vi "Increment Current Index.vi"(8 "Error In":errorcluster, 11 "reference in":refnum<class "Recipe.lvclass">) -> (0 "Error Out":errorcluster, 3 "reference out":refnum<class "Recipe.lvclass">)   [LabVIEW 2021, in "Recipe.lvclass"]
uses:
  Recipe.lvclass
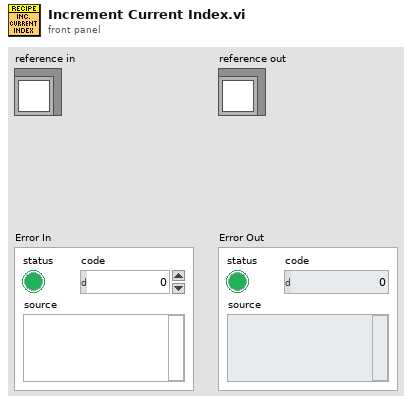
[diagram p1: front panel]
types:
  T1 = typedef "Recipe.lvclass/ObjectAttributes.ctl" = cluster{"Steps":refnum<class "Recipe Step.lvclass">[], "Current Info":cluster{"Current Index":u64}}
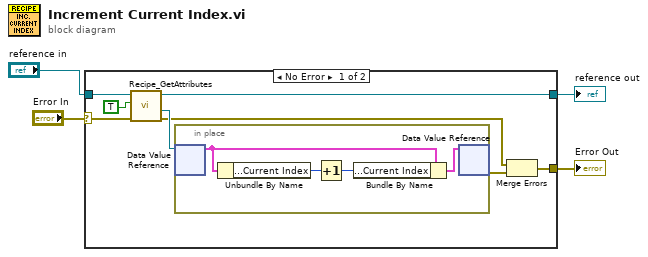
[diagram p0: block diagram]
diagram:
  n1 = case shown="No Error" "Error In" {
    selector: "Error In" -> [w11 w18]
    tunnel: [w8 w18] -> w3
    tunnel: [w9 w17] -> w1
    tunnel: "reference in" -> [w12 w17]
    frame No Error {
      n2 = call "Recipe_GetAttributes.vi"("Error In"=w11, "OnlyGetDvrReference(False)"=TRUE, "reference in"=w12) -> ("Error Out"=w6:errorcluster, "DataRef"=w7:refnum<data-value>, "reference out"=w9:refnum<class "Recipe.lvclass">)  [unwired: 5 in, 1 out]
      n3 = in-place {
        n4 = in-place-dvr #1(w7) -> (w15:T1)  [unwired: 1 out]
        n5 = Unbundle By Name(w15) -> ("Current Info.Current Index"=w14:u64)
        n6 = Increment(x=w14) -> (x+1=w13:u64)
        n7 = Bundle By Name(cluster=w15, "Current Info.Current Index"=w13) -> (w16:T1)
        n8 = in-place-dvr #1(w16) -> (w10:errorcluster)  [unwired: 1 out]
      }
      n9 = Merge Errors(w6, w10) -> (w8:errorcluster)
    }
    frame Error {
    }
  }
  "Error Out" <- w3
  "reference out" <- w1
